vi "DriveForTime.vi"() -> ()   [LabVIEW 2020]
uses:
  Framework/Robot Global Data.vi
panel:
  in  "NoWait":bool
  in  "Time":dbl
  in  "RightSpeed":dbl
  in  "LeftSpeed":dbl
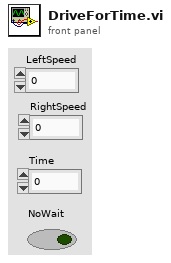
[diagram p1: front panel]
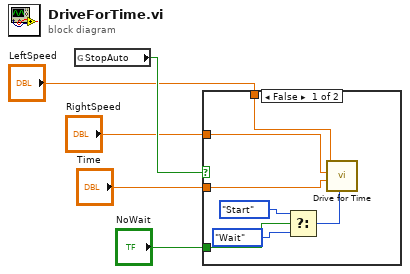
[diagram p0: block diagram]
diagram:
  n1 = global read "Robot Global Data.vi" "StopAuto"() -> (w5:bool)
  n2 = case shown="False" w5 {
    tunnel: "NoWait" -> [w11 _]
    tunnel: "Time" -> [w8 _]
    tunnel: "RightSpeed" -> [w7 _]
    tunnel: "LeftSpeed" -> [w6 _]
    frame False {
      n3 = Select(t=enum16{"Start", "Wait"}."Start" ("Synchronization"), s=w11, f=enum16{"Start", "Wait"}."Wait" ("Synchronization")) -> (s? t:f=w9:enum16{"Start", "Wait"})
      n4 = call "Drive for Time.vi"("Synchronization"=w9, "Seconds"=w8, "Right Speed"=w7, "Left Speed"=w6) -> ()  [unwired: 7 in, 1 out]
    }
    frame True {
    }
  }
